vi "9237_conversions.vi"(10 "offset_in":dbl[](array[numeric]), 11 "voltage_in":dbl[](array[numeric])) -> (0 "measured_axis_voltage":dbl[](array[numeric]), 3 "Array":dbl[](array[numeric]))   [LabVIEW 2019]
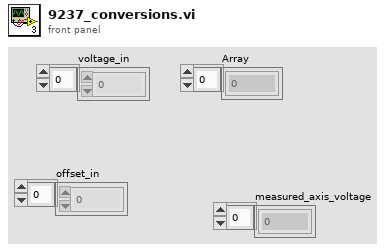
[diagram p1: front panel]
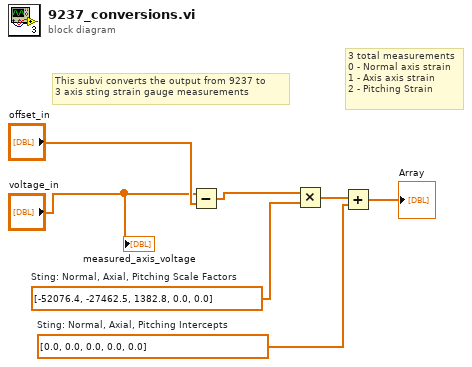
[diagram p0: block diagram]
diagram:
  w3 = dbl[] [0.0, 0.0, 0.0, 0.0, 0.0]  # Sting: Normal, Axial, Pitching Intercepts
  w4 = dbl[] [-52076.4, -27462.5, 1382.8, 0.0, 0.0]  # Sting: Normal, Axial, Pitching Scale Factors
  # "3 total measurements\n0 - Normal axis strain\n1 - Axis axis strain\n2 - Pitching Strain"
  # "This subvi converts the output from 9237 to \n3 axis sting strain gauge measurements"
  n1 = Subtract(x="voltage_in", y="offset_in") -> (x-y=w5:dbl[])
  n2 = Multiply(x=w5, y=w4) -> (x*y=w2:dbl[])
  n3 = Add(x=w2, y=w3) -> (x+y=→"Array":dbl[])
  "measured_axis_voltage" <- "voltage_in"
